vi "Read Frequency.vi"(8 "error in (no error)":errorcluster, 11 "Protocols in":refnum<class "Protocols.lvclass">) -> (0 "error out":errorcluster, 2 "Frequency":dbl, 3 "Protocols out":refnum<class "Protocols.lvclass">)   [LabVIEW 2020, in "I2C Controller.lvlib" / "Protocols.lvclass"]
uses:
  Protocols.lvclass
  Protocols.lvclass/Protocols.ctl
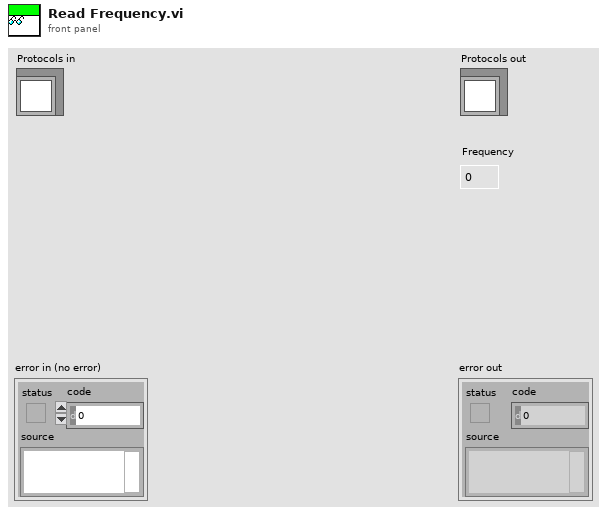
[diagram p1: front panel]
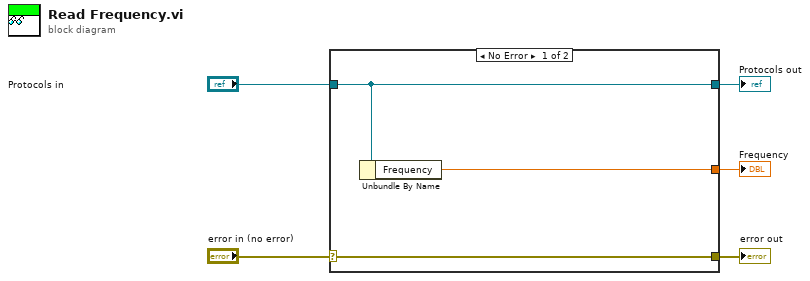
[diagram p0: block diagram]
diagram:
  n1 = case shown="No Error" "error in (no error)" {
    selector: "error in (no error)" -> [w8 w9]
    tunnel: [w8 w9] -> w4
    tunnel: [w7 w10] -> w2
    tunnel: "Protocols in" -> [w7 w10]
    tunnel: [w6 _] -> w1
    frame No Error {
      n2 = Unbundle By Name(w7) -> ("Frequency"=w6:dbl)
    }
    frame Error {
    }
  }
  "error out" <- w4
  "Protocols out" <- w2
  "Frequency" <- w1
